vi "Step Prescale Phase Factor.vi"(8 "error in (no error)":errorcluster, 9 "Step up? (false)":bool, 10 "Prescaler (Output AB)":i32(ring)=1 items=["Output AB"=1, "Output CD"=2, "Output EF"=3, "Output GH"=4], 11 "VISA resource name":refnum<visa-resource-name>) -> (0 "error out":errorcluster, 3 "VISA resource name out":refnum<visa-resource-name>, 4 "Device Errors":cluster{"code":i32, "Text":string}[](array[cluster]))   [LabVIEW 2014, in "Stanford Research DG645 - Driver.lvlib"]
doc: "Trigger Command: SPPH i,j\nInstrument Error Check\n\nStep prescale phase by the current step size in direction j. If j is true, then step up. If j is false, then step down. The parameter i selects the prescaler according to the following table:\n\ni Prescaler\n1 Output AB\n2 Output CD\n3 Output EF\n4 Output GH"
uses:
  Stanford Research DG645 - Driver.lvlib
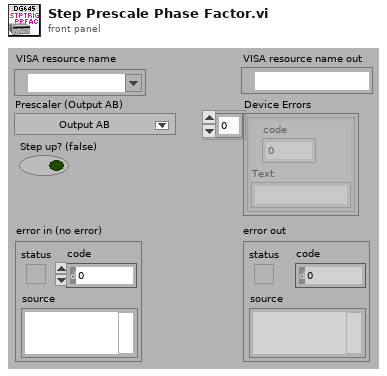
[diagram p1: front panel]
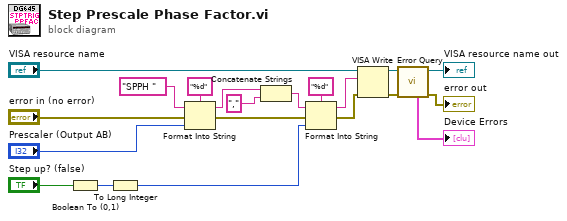
[diagram p0: block diagram]
diagram:
  n1 = Boolean To (0,1)(Boolean="Step up? (false)") -> (0, 1=w2:i16)
  n2 = To Long Integer(number=w2) -> (32bit integer=w1:i32)
  n3 = Format Into String(format string="%d", initial string="SPPH " ("command"), error in="error in (no error)", "Prescaler (Output AB)") -> (resulting string=w18:string, error out=w19:errorcluster)
  n4 = Concatenate Strings(w18, "," ("command")) -> (w13:string)
  n5 = Format Into String(format string="%d", initial string=w13, error in=w19, w1) -> (resulting string=w4:string, error out=w3:errorcluster)
  n6 = VISA Write(VISA resource name="VISA resource name", write buffer=w4, error in (no error)=w3) -> (VISA resource name out=w11:refnum<visa-resource-name>, error out=w8:errorcluster)  [unwired: 1 out]
  n7 = call "Error Query.vi"("error in (no error)"=w8, "VISA resource name"=w11) -> ("error out"=→"error out":errorcluster, "VISA resource name out"=→"VISA resource name out":refnum<visa-resource-name>, "Device Errors"=→"Device Errors":cluster{"code":i32, "Text":string}[])  [unwired: 7 in]
